vi "Generate PWM Pin Error.vi"(8 "Error In":errorcluster, 9 "Pin Number":u8, 10 "Board Type":T1) -> (0 "Error Out":errorcluster)   [LabVIEW 2011, in "LabVIEW Interface for ChipKit.lvlib"]
uses:
  LabVIEW Interface for ChipKit.lvlib
  Type Defs/Board Type.ctl
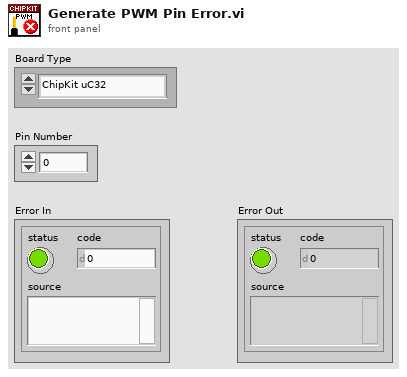
[diagram p1: front panel]
types:
  T1 = typedef "LabVIEW Interface for ChipKit.lvlib/Board Type.ctl" = enum16{"ChipKit uC32", "ChipKit Uno32", "ChipKit Max32"}
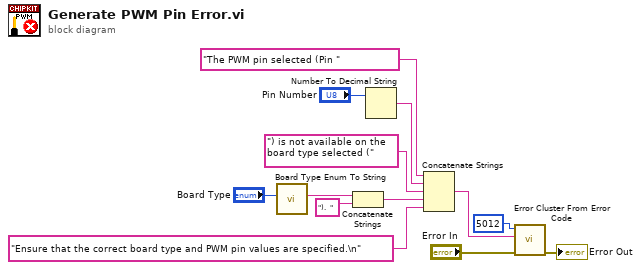
[diagram p0: block diagram]
diagram:
  n1 = call "Board Type Enum To String.vi"("Board Type"="Board Type") -> ("String"=w8:string)  [unwired: 10 in]
  n2 = Concatenate Strings(w8, ").  " ("string")) -> (w7:string)
  n3 = Number To Decimal String(number="Pin Number") -> (decimal integer string=w4:string)  [unwired: 1 in]
  n4 = Concatenate Strings("The PWM pin selected (Pin " ("source"), w4, ") is not available on the board type selected (" ("source"), w7, "Ensure that the correct board type and PWM pin values are specified.\n" ("source")) -> (w11:string)
  n5 = call <vilib>:"Error Cluster From Error Code.vi"("error in (no error)"="Error In", "error message (\"\")"=w11, "error code (0)"=5012) -> ("error out"=→"Error Out":errorcluster)  [unwired: 6 in]
